vi "DataLogger_GetFileName.vi"(8 "error in (no error)":errorcluster, 11 "Data Logger in":refnum<class "Data Logger.lvclass">) -> (0 "error out":errorcluster, 2 "File Name":string, 3 "Data Logger out":refnum<class "Data Logger.lvclass">)   [LabVIEW 2016, in "Data Logger.lvclass"]
uses:
  Data Logger.lvclass
  Data Logger.lvclass/Data Logger.ctl
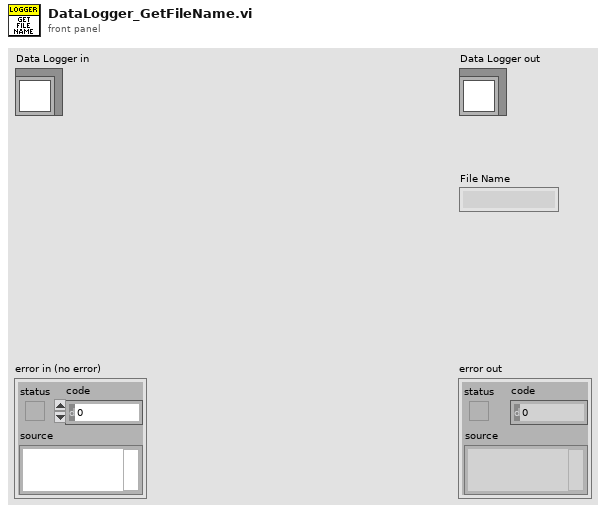
[diagram p1: front panel]
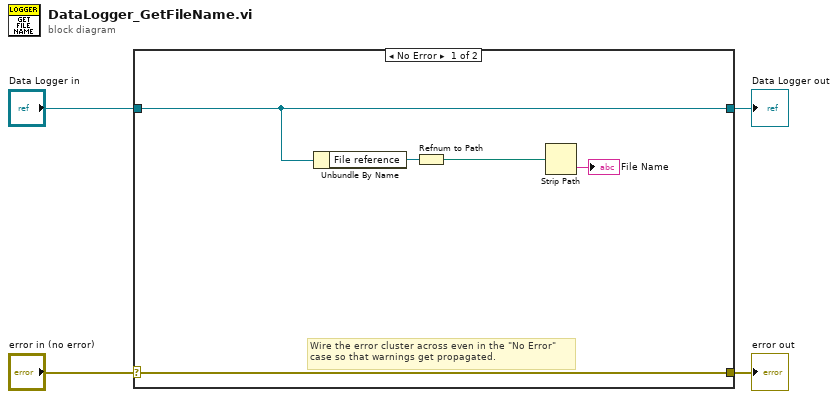
[diagram p0: block diagram]
diagram:
  n1 = case shown="No Error" "error in (no error)" {
    selector: "error in (no error)" -> [w9 w11]
    tunnel: [w9 w11] -> w3
    tunnel: [w8 w10] -> w1
    tunnel: "Data Logger in" -> [w8 w10]
    frame No Error {
      # "Wire the error cluster across even in the \"No Error\"\ncase so that warnings get propagated."
      n2 = Unbundle By Name(w8) -> ("File reference"=w6:refnum<file>)
      n3 = Refnum to Path(1:w6) -> (0:w5:path)
      n4 = Strip Path(path=w5) -> (name=→"File Name":string)  [unwired: 1 out]
    }
    frame Error {
    }
  }
  "error out" <- w3
  "Data Logger out" <- w1
